vi "Filter Channel Data.vi"(1 "Logger Parameters":T1) -> (0 "Filtered Data":dbl[][](array[numeric]))   [LabVIEW 2019, in "Telemetry Engine.lvlib"]
uses:
  Telemetry Engine.lvlib
  Types/Logger Data.ctl
  Types/Log File Properties.ctl
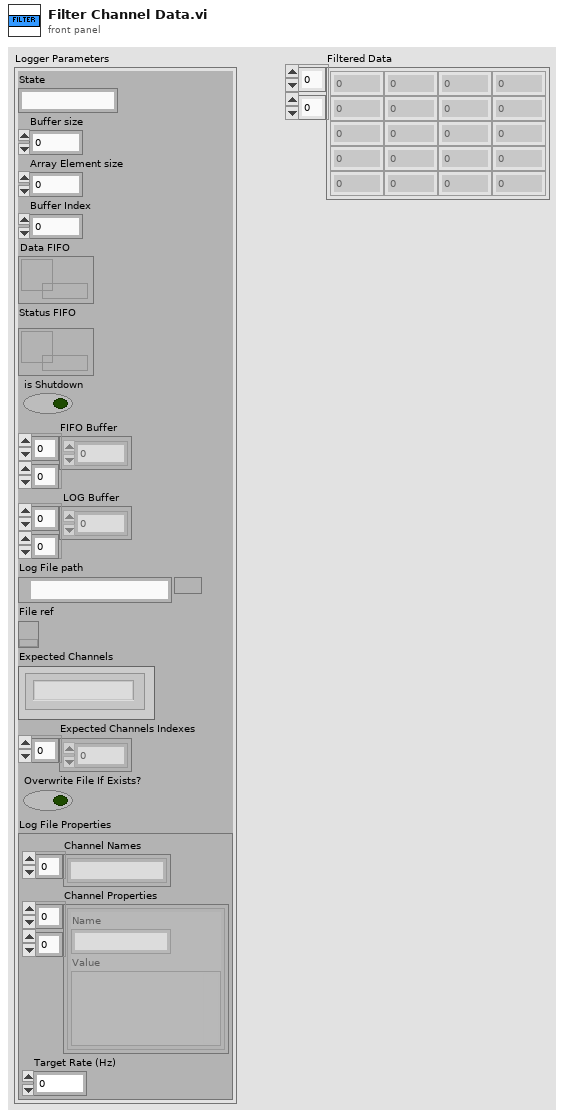
[diagram p1: front panel]
types:
  T1 = typedef "Telemetry Engine.lvlib/Logger Data.ctl" = cluster{"State":string, "Buffer size":i32, "Array Element size":i32, "Buffer Index":i32, "Data FIFO":refnum<k33>, "Status FIFO":refnum<k33>, "is Shutdown":bool, "FIFO Buffer":dbl[][], "LOG Buffer":dbl[][], "Log File path":path, "File ref":refnum<k34>, "Expected Channels":string[], "Expected Channels Indexes":i32[], "Overwrite File If Exists?":bool, "Log File Properties":T2}
  T2 = typedef "Telemetry Engine.lvlib/Log File Properties.ctl" = cluster{"Channel Names":string[], "Channel Properties":cluster{"Name":string, "Value":variant}[][], "Target Rate (Hz)":dbl}
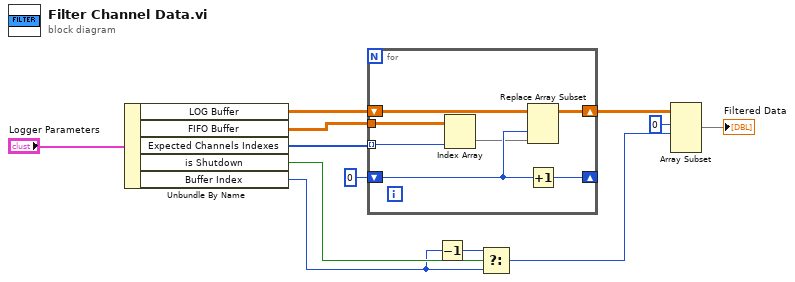
[diagram p0: block diagram]
diagram:
  n1 = Unbundle By Name("Logger Parameters") -> ("LOG Buffer"=w10:dbl[][], "FIFO Buffer"=w9:dbl[][], "Expected Channels Indexes"=w1:i32[], "is Shutdown"=w5:bool, "Buffer Index"=w4:i32)
  n2 = for {
    tunnel: w9 -> [w19]
    shift-right: [w15] -> w8
    shift-left: w10 -> [w17]
    shift-right: [w16] -> _
    shift-left: 0 -> [w18]
    tunnel: w1 -> [w13] mode=indexing
    n3 = Index Array(array=w19, index (col)=w13) -> (element=w14:dbl[])  [unwired: 1 in]
    n4 = Replace Array Subset(array=w17, new element=w14, index (col)=w18) -> (w15:dbl[][])  [unwired: 1 in]
    n5 = Increment(x=w18) -> (x+1=w16:i32)
  }
  n6 = Decrement(x=w4) -> (x-1=w6:i32)
  n7 = Select(t=w6, s=w5, f=w4) -> (s? t:f=w3:i32)
  n8 = Array Subset(array=w8, index (row)=0 ("index"), length (row)=w3) -> (→"Filtered Data":dbl[][])  [unwired: 2 in]
